vi "Get PolarPhase.vi"(8 "error in (no error)":errorcluster, 11 "TLCamera reference in":refnum<k24>) -> (0 "error out":errorcluster, 2 "PolarPhase":i32(ring) items=["PolarPhase0", "PolarPhase45", "PolarPhase90", "PolarPhase135"], 3 "TLCamera reference out":refnum<k24>)   [LabVIEW 2020]
uses:
  C:/GEECS/Developers Version/source/Device Drivers/Point Grey Camera/Library_X86/Thorlabs.TSI.TLCameraInterfaces.dll
  Point Grey Camera/Library_X86/Thorlabs.TSI.TLCameraInterfaces.dll
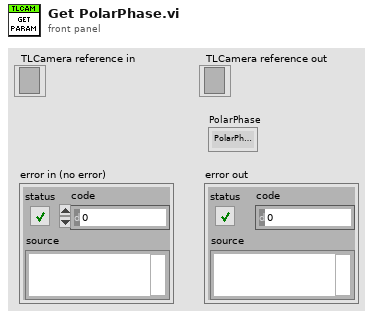
[diagram p1: front panel]
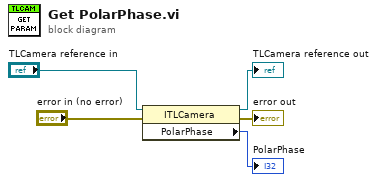
[diagram p0: block diagram]
diagram:
  n1 = property class="ITLCamera"(reference="TLCamera reference in", error in="error in (no error)") -> (reference out=→"TLCamera reference out":refnum<k24>, error out=→"error out":errorcluster, "PolarPhase"=→"PolarPhase":i32)
